vi "stringAddlength.vi"(10 "length":i32=4, 11 "Input":string) -> (1 "高低互换(4位)":string, 2 "Out":string)   [LabVIEW 2017]
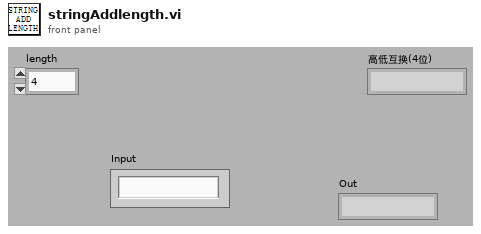
[diagram p1: front panel]
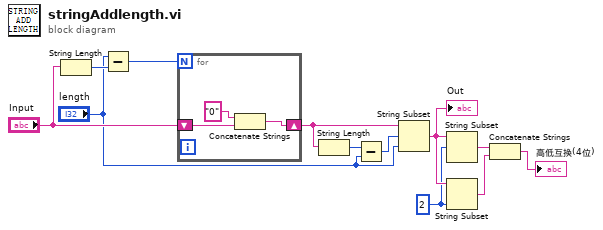
[diagram p0: block diagram]
diagram:
  w6 = 2 ("长度（剩余）")
  n1 = String Length(string="Input") -> (length=w12:i32)
  n2 = Subtract(x="length", y=w12) -> (x-y=w11:i32)
  n3 = for {
    N: w11 -> [_]
    shift-right: [w15] -> w10
    shift-left: "Input" -> [w14]
    n4 = Concatenate Strings("0" ("字符串"), w14) -> (w15:string)
  }
  n5 = String Length(string=w10) -> (length=w9:i32)
  n6 = Subtract(x=w9, y="length") -> (x-y=w8:i32)
  n7 = String Subset(string=w10, offset (0)=w8, length (rest)="length") -> (substring=w7:string)
  "Out" <- w7
  n8 = String Subset(string=w7, offset (0)=w6) -> (substring=w4:string)  [unwired: 1 in]
  n9 = String Subset(string=w7, length (rest)=w6) -> (substring=w5:string)  [unwired: 1 in]
  n10 = Concatenate Strings(w4, w5) -> (→"高低互换(4位)":string)
